vi "array to IMAQ.vi"(8 "error in (no error)":errorcluster, 11 "Cascade in":refnum<class "Cascade.lvclass">) -> (0 "error out":errorcluster, 3 "Cascade out":refnum<class "Cascade.lvclass">)   [LabVIEW 2012, in "Cascade.lvclass"]
uses:
  Cascade.lvclass
  Cascade.lvclass/Cascade.ctl
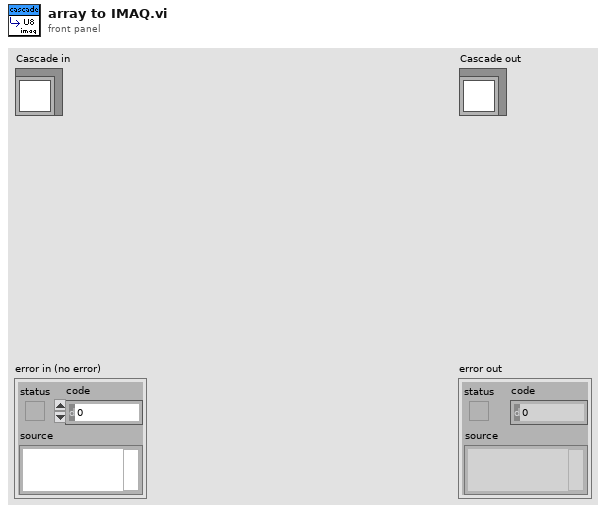
[diagram p1: front panel]
types:
  T1 = typedef "IMAQ Image.ctl" = refnum<image>
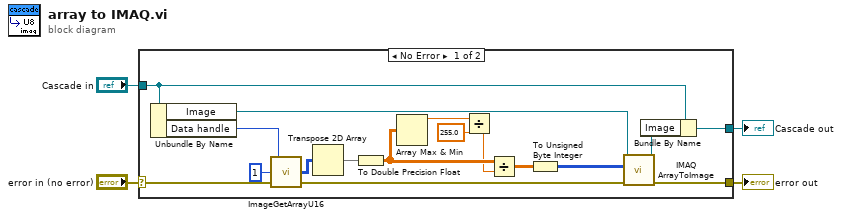
[diagram p0: block diagram]
diagram:
  n1 = case shown="No Error" "error in (no error)" {
    selector: "error in (no error)" -> [w21 w23]
    tunnel: [w15 w23] -> w3
    tunnel: [w17 w22] -> w1
    tunnel: "Cascade in" -> [w18 w22]
    frame No Error {
      n2 = Unbundle By Name(w18) -> ("Image"=w13:T1, "Data handle"=w20:u32)
      n3 = call <userlib>:"ImageGetArrayU16.vi"("error in"=w21, "Z position"=u32 1, "Image Handle"=w20) -> ("error out"=w16:errorcluster, "Array uint 16"=w14:u16[][])  [unwired: 1 out]
      n4 = Transpose 2D Array(2D array=w14) -> (transposed array=w11:u16[][])
      n5 = To Double Precision Float(number=w11) -> (double precision float=w10:dbl[][])
      n6 = Array Max & Min(array=w10) -> (max value=w9:dbl)  [unwired: 3 out]
      n7 = Divide(x=w9, y=255.0) -> (x/y=w7:dbl)
      n8 = Divide(x=w10, y=w7) -> (x/y=w6:dbl[][])
      n9 = To Unsigned Byte Integer(number=w6) -> (unsigned 8bit integer=w5:u8[][])
      n10 = call "IMAQ ArrayToImage"("error in (no error)"=w16, "Image Pixels (U8)"=w5, "Image"=w13) -> ("error out"=w15:errorcluster, "Image Out"=w12:T1)  [unwired: 7 in]
      n11 = Bundle By Name(cluster=w18, "Image"=w12) -> (w17:refnum<class "Cascade.lvclass">)
    }
    frame Error {
    }
  }
  "error out" <- w3
  "Cascade out" <- w1
